vi "SnoTrapazoidalTrajectory.vi"(1 "Straight or Turn":bool=TRUE, 2 "Ramp_Up/Down_Time (sec.)":dbl=1.0, 3 "Drive Forward/Reverse":bool=TRUE, 4 "error in":errorcluster, 5 "RobotDriveDevRef":T1={"DevStatus"={"status"=FALSE, "code"=0, "source"=""}, "Motors[]"=[], "Square Inputs"=FALSE, "Max Output"=1.0}, 6 "Max Speed":dbl, 7 "Seconds for Traversal":dbl) -> (0 "error out":errorcluster)   [LabVIEW 2014]
uses:
  <vilib>/Rock Robotics/WPI/RobotDrive/WPI_RobotDriveDevRef.ctl
  <vilib>/Rock Robotics/WPI/MotorControl/WPI_MotorControlDeviceRef.ctl
  <vilib>/Rock Robotics/WPI/MotorControl/WPI_MotorControlType.ctl
  <vilib>/Rock Robotics/SystemInterfaces/Typedef/FPGA_TypedefDigitalModule.ctl
  <vilib>/Rock Robotics/SystemInterfaces/DIO/FPGA_DIOPWMChannel.ctl
  <vilib>/Rock Robotics/WPI/PWM/WPI_PWMDeadband.ctl
  <vilib>/Rock Robotics/WPI/CAN/Jaguar/SubVIs/WPI_CANJaguar_ControlMode.ctl
  <vilib>/Rock Robotics/WPI/CAN/TalonSRX/WPI_CANTalonSRX_APIControlMode.ctl
  <vilib>/Rock Robotics/WPI/PWM/WPI_PWMTransform_ConPane.ctl
panel:
  out "1/2 Traversal Time (mSec)":u32
  out "Relative Time (Sec)":dbl
  out "Motor Command":dbl
  out "Ramp Up/Down Time (mSec.)":u32
  out "Waveform Chart":dbl(graph)
  out "Slope":dbl
  out "Ramp Up/Down":bool
  out "Relative End Time":u32
  out "Relative Time (mSec)":u32
  out "Tmer value (mSec)":u32
  out "End Time (mSec)":u32
  out "Start Time (mSec)":u32
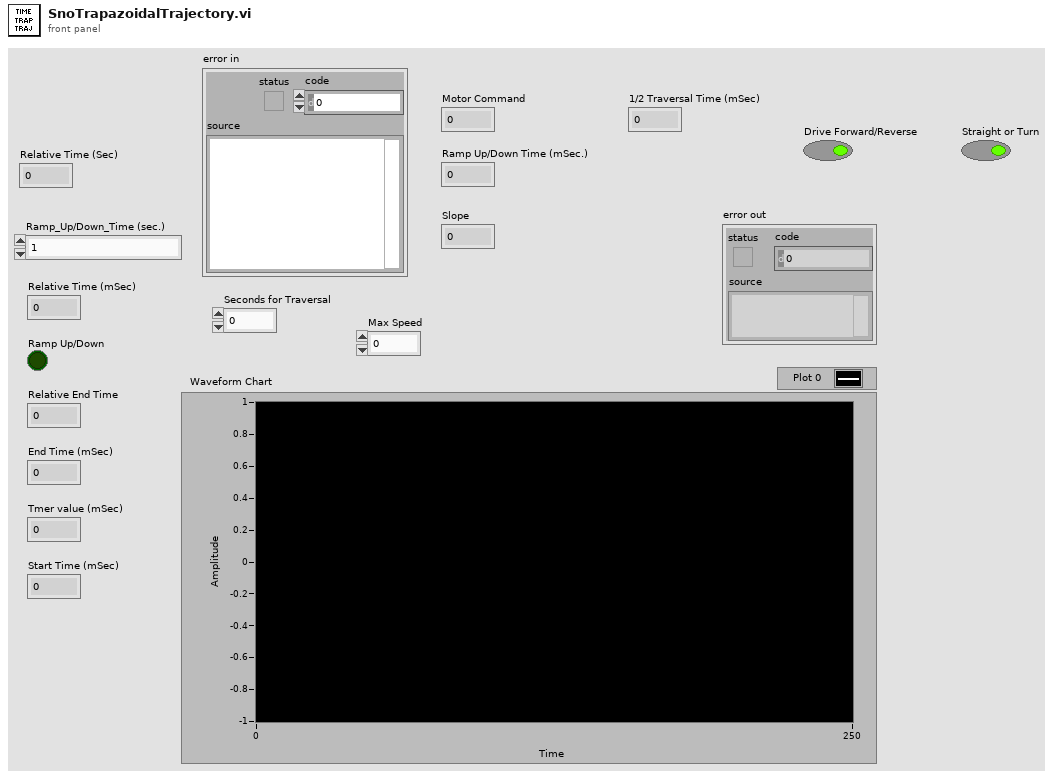
[diagram p1: front panel]
types:
  T1 = typedef "WPI_RobotDriveDevRef.ctl" = cluster{"DevStatus":errorcluster, "Motors[]":T2[], "Square Inputs":bool, "Max Output":dbl}
  T2 = typedef "WPI_MotorControlDeviceRef.ctl" = cluster{"DeviceStatus":errorcluster, "Type":T3, "PWM":cluster{"Controller":T4, "PWM Channel":T5, "DeadBand":T6}, "CAN":cluster{"Device Number":u8, "Control Mode":T7, "Semaphore":T8, "Max Vout":dbl, "TalonSRX Control Mode":T9}, "Invert":bool, "TransformRef":T10, "InvTransformRef":T10}
  T3 = typedef "WPI_MotorControlType.ctl" = enum16{"PWM", "CAN", "CANTalonSRX"}
  T4 = typedef "FPGA_TypedefDigitalModule.ctl" = enum16{"Controller 1"}
  T5 = typedef "FPGA_DIOPWMChannel.ctl" = enum8{"PWM 0", "PWM 1", "PWM 2", "PWM 3", "PWM 4", "PWM 5", "PWM 6", "PWM 7", "PWM 8", "PWM 9", "PWM MXP 0", "PWM MXP 1", "PWM MXP 2", "PWM MXP 3", "PWM MXP 4", "PWM MXP 5", "PWM MXP 6", "PWM MXP 7", "PWM MXP 8", "PWM MXP 9", "Invalid"}
  T6 = typedef "WPI_PWMDeadband.ctl" = cluster{"Name":string, "maxPositivePwm":i32, "minPositivePwm":i32, "centerPwm":i32, "maxNegativePwm":i32, "minNegativePwm":i32, "angularRange":u16}
  T7 = typedef "WPI_CANJaguar_ControlMode.ctl" = enum8{"Percent VBus", "Current", "Speed", "Position", "Voltage"}
  T8 = typedef "Semaphore RefNum" = refnum<k1>
  T9 = typedef "WPI_CANTalonSRX_APIControlMode.ctl" = enum8{"Percent VBus", "Speed", "Position", "Slave", "Unchanged / Invalid"}
  T10 = typedef "WPI_PWMTransform_ConPane.ctl" = refnum<vi>
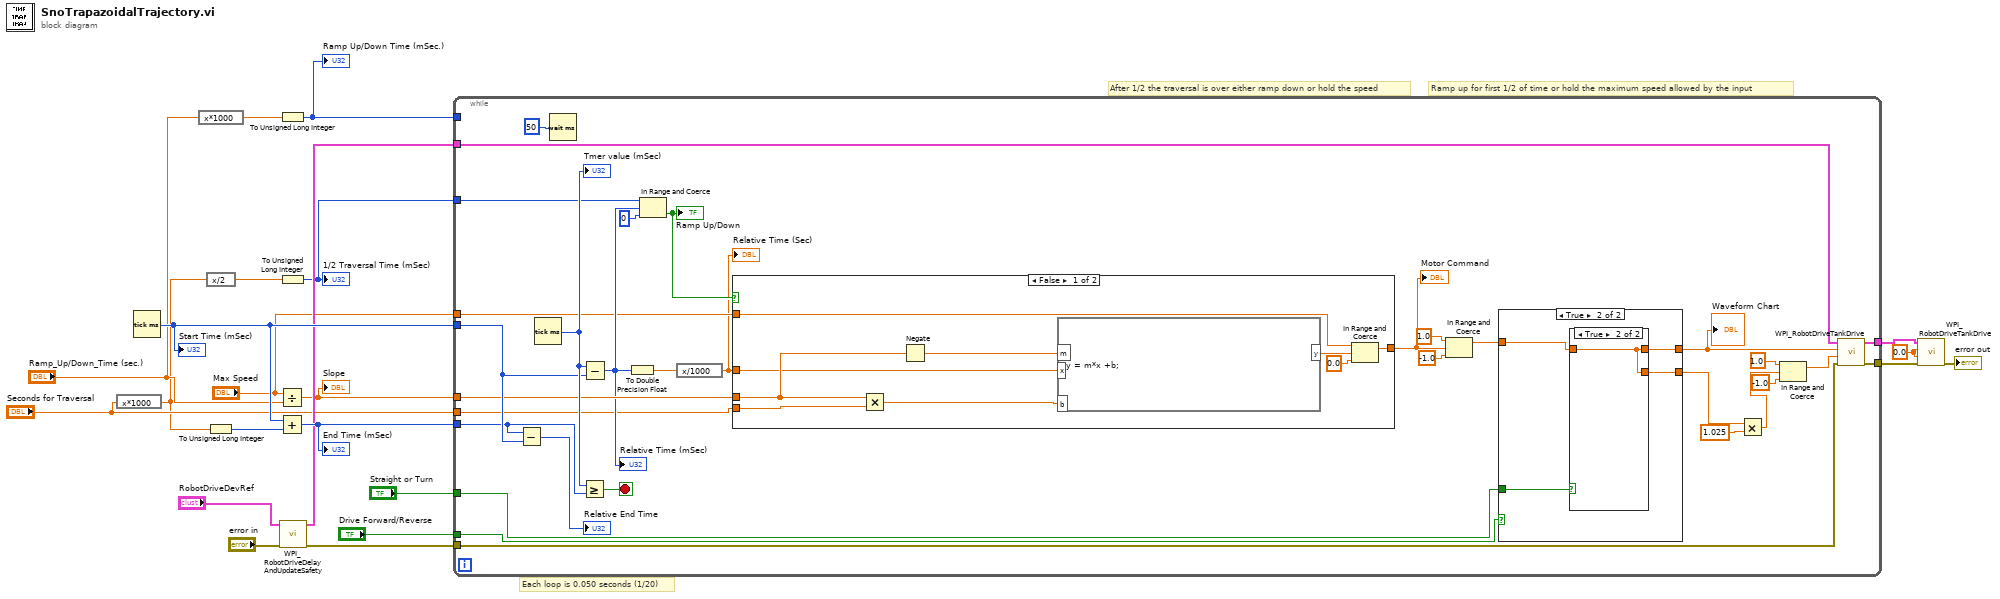
[diagram p0: block diagram]
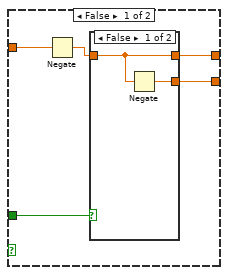
[diagram p2: hidden frame]
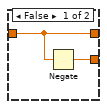
[diagram p4: hidden frame]
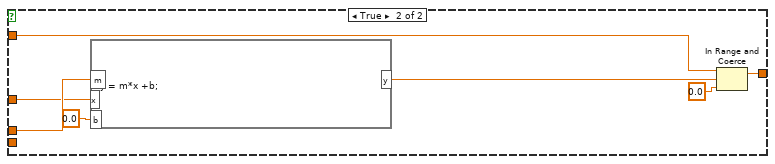
[diagram p5: hidden frame]
diagram:
  w19 = 0.0 ("Left axis value")
  # "After 1/2 the traversal is over either ramp down or hold the speed"
  # "Ramp up for first 1/2 of time or hold the maximum speed allowed by the input"
  # "Each loop is 0.050 seconds (1/20)"
  n1 = expression code="x*1000"("Seconds for Traversal") -> (w3:dbl)
  n2 = Tick Count (ms)() -> (millisecond timer value=w21:u32)
  "Start Time (mSec)" <- w21
  n3 = expression code="x*1000"("Ramp_Up/Down_Time (sec.)") -> (w4:dbl)
  n4 = expression code="x/2"(w3) -> (w7:dbl)
  n5 = To Unsigned Long Integer(number=w3) -> (unsigned 32bit integer=w11:u32)
  n6 = Divide(x="Max Speed", y="Ramp_Up/Down_Time (sec.)") -> (x/y=w9:dbl)
  "Slope" <- w9
  n7 = Add(x=w21, y=w11) -> (x+y=w20:u32)
  "End Time (mSec)" <- w20
  n8 = To Unsigned Long Integer(number=w4) -> (unsigned 32bit integer=w13:u32)
  "Ramp Up/Down Time (mSec.)" <- w13
  n9 = To Unsigned Long Integer(number=w7) -> (unsigned 32bit integer=w10:u32)
  "1/2 Traversal Time (mSec)" <- w10
  n10 = call <vilib>:"WPI_RobotDriveDelayAndUpdateSafety.vi"("error in (no error)"="error in", "RobotDriveDevRef"="RobotDriveDevRef") -> ("error out"=w14:errorcluster, "RobotDriveDevRef 2"=w17:T1)  [unwired: 8 in]
  n11 = while {
    tunnel: w20 -> [w51]
    tunnel: w21 -> [w52]
    tunnel: w17 -> [w40]
    tunnel: [w38] -> w22
    tunnel: w14 -> [w41]
    tunnel: [w39] -> w16
    tunnel: w13 -> [_]
    tunnel: w10 -> [w48]
    tunnel: w9 -> [w47]
    tunnel: "Max Speed" -> [w45]
    tunnel: "Seconds for Traversal" -> [w37]
    tunnel: "Drive Forward/Reverse" -> [w32]
    tunnel: "Straight or Turn" -> [w29]
    stop <- w54 stop-if-true
    n12 = Subtract(x=w51, y=w52) -> (x-y=→"Relative End Time":u32)
    n13 = Tick Count (ms)() -> (millisecond timer value=w53:u32)
    "Tmer value (mSec)" <- w53
    n14 = Wait (ms)(milliseconds to wait=u32 50) -> ()  [unwired: 1 out]
    n15 = Greater Or Equal?(x=w53, y=w51) -> (x >= y?=w54:bool)
    n16 = Subtract(x=w53, y=w52) -> (x-y=w46:u32)
    "Relative Time (mSec)" <- w46
    n17 = To Double Precision Float(number=w46) -> (double precision float=w34:dbl)
    n18 = In Range and Coerce(upper limit=w48, x=w46, lower limit=u32 0) -> (In Range?=w35:bool)  [unwired: 1 out]
    "Ramp Up/Down" <- w35
    n19 = expression code="x/1000"(w34) -> (w33:dbl)
    "Relative Time (Sec)" <- w33
    n20 = case shown="False" w35 {
      tunnel: w47 -> [w77 w85]
      tunnel: w33 -> [w74 w79]
      tunnel: w45 -> [w72 w81]
      tunnel: [w71 w80] -> w42
      tunnel: w37 -> [w76 _]
      frame False {
        n21 = Multiply(x=w77, y=w76) -> (x*y=w75:dbl)
        n22 = Negate(x=w77) -> (-x=w78:dbl)
        n23 = formula code="y = m*x +b;"("m"=w78, "x"=w74, "b"=w75) -> ("y"=w70:dbl)
        n24 = In Range and Coerce(upper limit=w72, x=w70, lower limit=0.0 ("upper limit")) -> (coerced(x)=w71:dbl)  [unwired: 1 out]
      }
      frame True {
        n25 = formula code="y = m*x +b;"("m"=w85, "x"=w79, "b"=0.0 ("input variable")) -> ("y"=w83:dbl)
        n26 = In Range and Coerce(upper limit=w81, x=w83, lower limit=0.0) -> (coerced(x)=w80:dbl)  [unwired: 1 out]
      }
    }
    "Motor Command" <- w42
    n27 = In Range and Coerce(upper limit=1.0, x=w42, lower limit=-1.0) -> (coerced(x)=w31:dbl)  [unwired: 1 out]
    n28 = case shown="True" w32 {
      tunnel: w31 -> [w59 w63]
      tunnel: [w56 w64] -> w25
      tunnel: [w57 w65] -> w30
      tunnel: w29 -> [w55 w66]
      frame False {
        n29 = Negate(x=w59) -> (-x=w58:dbl)
        n30 = case shown="False" w55 {
          tunnel: [w61 w62] -> w57
          tunnel: [w60 w62] -> w56
          tunnel: w58 -> [w61 w62]
          frame False {
            n31 = Negate(x=w61) -> (-x=w60:dbl)
          }
          frame True {
          }
        }
      }
      frame True {
        n32 = case shown="True" w66 {
          tunnel: [w68 w69] -> w65
          tunnel: [w67 w69] -> w64
          tunnel: w63 -> [w68 w69]
          frame False {
            n33 = Negate(x=w68) -> (-x=w67:dbl)
          }
          frame True {
          }
        }
      }
    }
    "Waveform Chart" <- w30
    n34 = Multiply(x=w25, y=1.025) -> (x*y=w23:dbl)
    n35 = In Range and Coerce(upper limit=1.0, x=w23, lower limit=-1.0) -> (coerced(x)=w26:dbl)  [unwired: 1 out]
    n36 = call <vilib>:"WPI_RobotDriveTankDrive.vi"("error in (no error)"=w41, "Right axis value"=w26, "Left axis value"=w30, "RobotDriveDevRef"=w40) -> ("error out"=w38:errorcluster, "RobotDriveDevRef"=w39:T1)  [unwired: 5 in, 1 out]
  }
  n37 = call <vilib>:"WPI_RobotDriveTankDrive.vi"("error in (no error)"=w22, "Right axis value"=w19, "Left axis value"=w19, "RobotDriveDevRef"=w16) -> ("error out"=→"error out":errorcluster)  [unwired: 5 in, 2 out]
